vi "HTTP Dynamic VIs.vi"   [LabVIEW 2011, in "NI_InternetTK_Core_VIs.lvlib"]
uses:
  <vilib>/addons/internet/NI_InternetTK_Core_VIs.lvlib
panel:
  # "This VI and its subVIs contain all the VIs needed for the HTTP Server\nto support its basic operation, including serving images of VI panels.\nYou can \"Save with Options...\" this VI in order to build an executable\nwith an embeded HTTP server. \n\nThis VI does not include all the VIs needed for CGI operation.\n\nIf you build an executable from these VIs, make sure to ship the DLLs\nin the /usr.lib/internet/image/ directory with the executable."
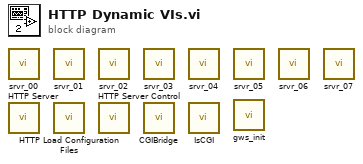
[diagram p0: block diagram]
diagram:
  n1 = call <vilib>:"srvr_00.vi"() -> ()  [unwired: 1 out]
  n2 = call "HTTP Server"() -> ()  [unwired: 1 out]
  n3 = call <vilib>:"srvr_01.vi"() -> ()  [unwired: 1 out]
  n4 = call <vilib>:"HTTP Load Configuration Files.vi"() -> ()  [unwired: 2 in, 6 out]
  n5 = call <vilib>:"srvr_02.vi"() -> ()  [unwired: 1 out]
  n6 = call <vilib>:"HTTP Server Control.vi"() -> ()  [unwired: 3 in, 5 out]
  n7 = call <vilib>:"srvr_03.vi"() -> ()  [unwired: 1 out]
  n8 = call <vilib>:"CGIBridge.vi"() -> ()  [unwired: 5 in, 7 out]
  n9 = call <vilib>:"srvr_04.vi"() -> ()  [unwired: 1 out]
  n10 = call <vilib>:"IsCGI.vi"() -> ()  [unwired: 1 in, 11 out]
  n11 = call <vilib>:"srvr_05.vi"() -> ()  [unwired: 1 out]
  n12 = call <vilib>:"gws_init.vi"() -> ()  [unwired: 1 out]
  n13 = call <vilib>:"srvr_06.vi"() -> ()  [unwired: 1 out]
  n14 = call <vilib>:"srvr_07.vi"() -> ()  [unwired: 1 out]
